vi "Create PPL.vi"(11 "error in (no error)":errorcluster) -> (15 "error out":errorcluster)   [LabVIEW 2021, in "G Plug-in Migrator.lvlib"]
uses:
  G Plug-in Migrator.lvlib
  Generator/_InstrumentStudio Plug-In Editor/NI_AB_API_PPL_Extensions/NI_AB_API_PPL_Extensions.lvclass
  Migrator Reusables/Migrator Reusables.lvlib
  Path Functions/Path Functions.lvlib
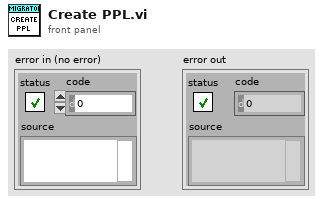
[diagram p1: front panel]
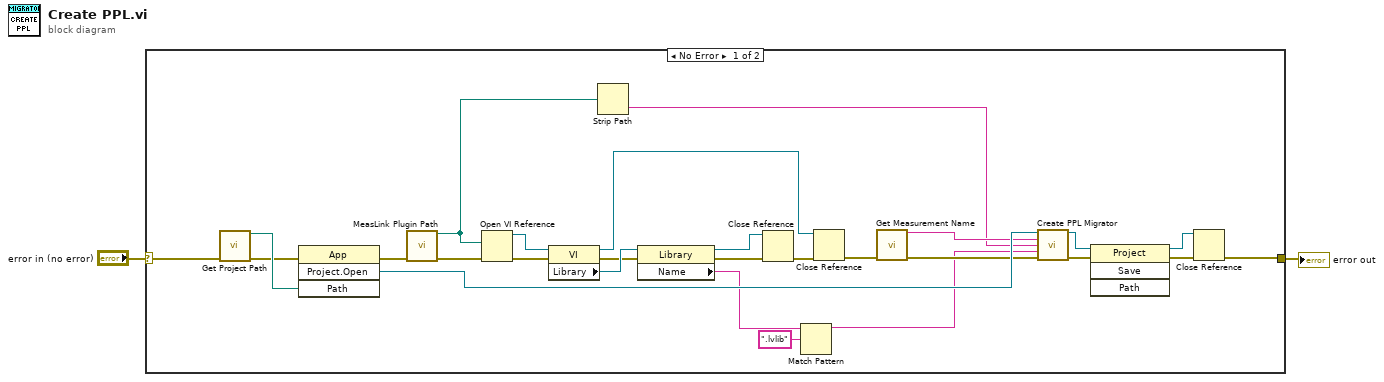
[diagram p0: block diagram]
diagram:
  n1 = case shown="No Error" "error in (no error)" {
    selector: "error in (no error)" -> [w27 w30]
    tunnel: [w8 w30] -> w2
    frame No Error {
      n2 = call "Get Project Path.vi"("error in (no error)"=w27) -> ("Project Path Out"=w29:path, "error out"=w28:errorcluster)  [unwired: 13 in]
      n3 = invoke class="App" method="Project.Open"(error in=w28, "Path"=w29) -> (error out=w5:errorcluster, "Project:Open"=w26:refnum<vi>)  [unwired: 2 in, 2 out]
      n4 = call "MeasLink Plugin Path.vi"("error in (no error)"=w5) -> ("New Code Module"=w7:path, "error out"=w6:errorcluster)  [unwired: 2 in, 11 out]
      n5 = Open VI Reference(vi path=w7, error in (no error)=w6) -> (vi reference=w24:refnum<vi>, error out=w15:errorcluster)  [unwired: 4 in]
      n6 = property class="VI"(reference=w24, error in=w15) -> (reference out=w16:refnum<vi>, error out=w14:errorcluster, "Library"=w23:refnum<vi>)
      n7 = Strip Path(path=w7) -> (name=w20:string)  [unwired: 1 out]
      n8 = property class="Library"(reference=w23, error in=w14) -> (reference out=w18:refnum<vi>, error out=w19:errorcluster, "Name"=w22:string)
      n9 = Close Reference(reference=w18, error in (no error)=w19) -> (error out=w17:errorcluster)
      n10 = Match Pattern(string=w22, regular expression=".lvlib") -> (before substring=w4:string)  [unwired: 1 in, 3 out]
      n11 = Close Reference(reference=w16, error in (no error)=w17) -> (error out=w13:errorcluster)
      n12 = call "Get Measurement Name.vi"("error in (no error)"=w13) -> ("Name Out"=w25:string, "error out"=w21:errorcluster)  [unwired: 13 in]
      n13 = call "Create PPL Migrator.vi"("Project Refnum"=w26, "Plug-in name"=w25, "Main VI Name"=w20, "Library name"=w4, "error in (no error)"=w21) -> ("project ref out"=w12:refnum<vi>, "error out"=w11:errorcluster)  [unwired: 8 in, 1 out]
      n14 = invoke class="Project" method="Save"(reference=w12, error in=w11) -> (reference out=w9:refnum<vi>, error out=w10:errorcluster)  [unwired: 2 in, 2 out]
      n15 = Close Reference(reference=w9, error in (no error)=w10) -> (error out=w8:errorcluster)
    }
    frame Error {
    }
  }
  "error out" <- w2
